vi "Frame Data FGV [Body Index].vi"(6 "Command":enum16{"Get", "Initialize"}(ring), 8 "error in (no error)":errorcluster, 10 "FrameDescription":T1) -> (0 "error out":errorcluster, 2 "Array":u8[](array[numeric]))   [LabVIEW 2014]
uses:
  controls/FrameDescription.ctl
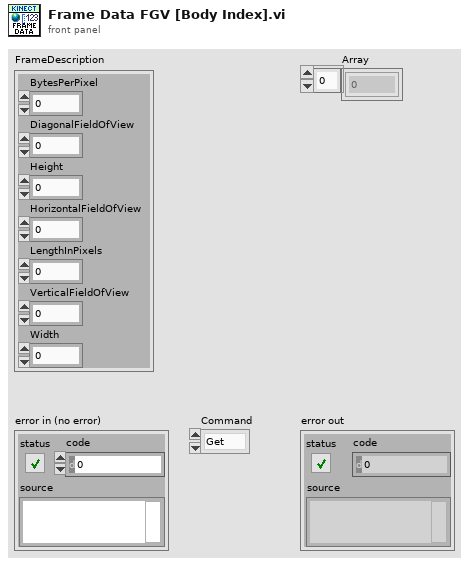
[diagram p1: front panel]
types:
  T1 = typedef "FrameDescription.ctl" = cluster{"BytesPerPixel":u32, "DiagonalFieldOfView":sgl, "Height":i32, "HorizontalFieldOfView":sgl, "LengthInPixels":u32, "VerticalFieldOfView":sgl, "Width":i32}
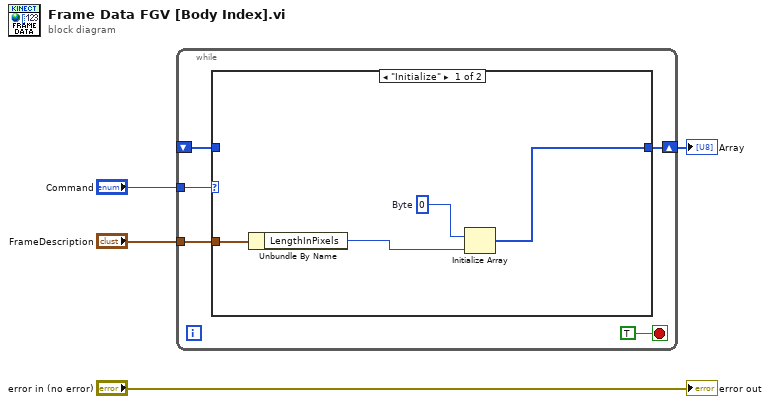
[diagram p0: block diagram]
diagram:
  n1 = while {
    tunnel: "Command" -> [w9]
    tunnel: "FrameDescription" -> [w8]
    shift-right: [w7] -> w1
    shift-left: _ -> [w6]
    stop <- TRUE stop-if-true
    n2 = case shown="\"Initialize\"" w9 {
      tunnel: w8 -> [w12 _]
      tunnel: [w11 w14] -> w7
      tunnel: w6 -> [_ w14]
      frame "Initialize" {
        w13 = u8 0  # Byte
        n3 = Unbundle By Name(w12) -> ("LengthInPixels"=w10:u32)
        n4 = Initialize Array(w13, w10) -> (w11:u8[])
      }
      frame "Get", Default {
      }
    }
  }
  "Array" <- w1
  "error out" <- "error in (no error)"
